vi "enable disable channel for saving.vi"() -> ()   [LabVIEW 2018]
uses:
  <vilib>/Utility/miscctls.llb/LVPointTypeDef.ctl
  <vilib>/Utility/file.llb/Write Delimited Spreadsheet (I64).vi
  <vilib>/Utility/file.llb/Read Delimited Spreadsheet (I64).vi
panel:
  out "size(s) 2":i32=165
  in  "Home Button":bool
  in  "Save Button":bool
  in  "Tab Control":enum32{"Page 1", "Page 2"}(tab)
  in  "Channel 1":cluster{"Enable":bool, "Channel Name":string}={"Enable"=TRUE, "Channel Name"="Time"}
  in  "Channel 2":cluster{"Enable":bool, "Channel Name":string}={"Enable"=TRUE, "Channel Name"="Throttle % "}
  in  "Channel 3":cluster{"Enable":bool, "Channel Name":string}={"Enable"=TRUE, "Channel Name"="Set Speed"}
  in  "Channel 4":cluster{"Enable":bool, "Channel Name":string}={"Enable"=TRUE, "Channel Name"="Speed Summary"}
  in  "Channel 5":cluster{"Enable":bool, "Channel Name":string}={"Enable"=TRUE, "Channel Name"="Torque Summary"}
  in  "Channel 6":cluster{"Enable":bool, "Channel Name":string}={"Enable"=TRUE, "Channel Name"="Power"}
  in  "Channel 7":cluster{"Enable":bool, "Channel Name":string}={"Enable"=TRUE, "Channel Name"="Gear Ratio"}
  in  "Channel 8":cluster{"Enable":bool, "Channel Name":string}={"Enable"=TRUE, "Channel Name"="H Dyno Speed"}
  in  "Channel 9":cluster{"Enable":bool, "Channel Name":string}={"Enable"=TRUE, "Channel Name"="H Dyno Torque"}
  in  "Channel 10":cluster{"Enable":bool, "Channel Name":string}={"Enable"=TRUE, "Channel Name"="L Speed"}
  in  "Channel 11":cluster{"Enable":bool, "Channel Name":string}={"Enable"=TRUE, "Channel Name"="R Speed"}
  in  "Channel 12":cluster{"Enable":bool, "Channel Name":string}={"Enable"=TRUE, "Channel Name"="H Speed"}
  in  "Channel 13":cluster{"Enable":bool, "Channel Name":string}={"Enable"=TRUE, "Channel Name"="L Torque "}
  in  "Channel 14":cluster{"Enable":bool, "Channel Name":string}={"Enable"=TRUE, "Channel Name"="R Torque "}
  in  "Channel 15":cluster{"Enable":bool, "Channel Name":string}={"Enable"=TRUE, "Channel Name"="H Torque "}
  in  "Channel 16":cluster{"Enable":bool, "Channel Name":string}={"Enable"=TRUE, "Channel Name"="T_Oil Gallery"}
  in  "Channel 17":cluster{"Enable":bool, "Channel Name":string}={"Enable"=TRUE, "Channel Name"="T_Coolant_Out"}
  in  "Channel 18":cluster{"Enable":bool, "Channel Name":string}={"Enable"=TRUE, "Channel Name"="T_Coolant_In"}
  in  "Channel 19":cluster{"Enable":bool, "Channel Name":string}={"Enable"=TRUE, "Channel Name"="T_Oil Pan_Out"}
  in  "Channel 20":cluster{"Enable":bool, "Channel Name":string}={"Enable"=TRUE, "Channel Name"="T_Intercooler_In"}
  in  "Channel 21":cluster{"Enable":bool, "Channel Name":string}={"Enable"=TRUE, "Channel Name"="T_Intercooler_Out"}
  in  "Channel 22":cluster{"Enable":bool, "Channel Name":string}={"Enable"=TRUE, "Channel Name"="T_Exhaust_Tail pipe"}
  in  "Channel 23":cluster{"Enable":bool, "Channel Name":string}={"Enable"=TRUE, "Channel Name"="T_frt winding"}
  in  "Channel 24":cluster{"Enable":bool, "Channel Name":string}={"Enable"=TRUE, "Channel Name"="T_Stator Core"}
  in  "Channel 25":cluster{"Enable":bool, "Channel Name":string}={"Enable"=TRUE, "Channel Name"="T_Before Cat"}
  in  "Channel 26":cluster{"Enable":bool, "Channel Name":string}={"Enable"=TRUE, "Channel Name"="TC11"}
  in  "Channel 27":cluster{"Enable":bool, "Channel Name":string}={"Enable"=TRUE, "Channel Name"="TC12"}
  in  "Channel 28":cluster{"Enable":bool, "Channel Name":string}={"Enable"=TRUE, "Channel Name"="TC13"}
  in  "Channel 29":cluster{"Enable":bool, "Channel Name":string}={"Enable"=TRUE, "Channel Name"="TC14"}
  in  "Channel 30":cluster{"Enable":bool, "Channel Name":string}={"Enable"=TRUE, "Channel Name"="TC15"}
  in  "Channel 31":cluster{"Enable":bool, "Channel Name":string}={"Enable"=TRUE, "Channel Name"="TC16"}
  in  "Channel 32":cluster{"Enable":bool, "Channel Name":string}={"Enable"=TRUE, "Channel Name"="P_Oil Gallery"}
  in  "Channel 33":cluster{"Enable":bool, "Channel Name":string}={"Enable"=TRUE, "Channel Name"="P_Coolant_IN"}
  in  "Channel 34":cluster{"Enable":bool, "Channel Name":string}={"Enable"=TRUE, "Channel Name"="P_Coolant_OUT"}
  in  "Channel 35":cluster{"Enable":bool, "Channel Name":string}={"Enable"=TRUE, "Channel Name"="P_Intercooler_In"}
  in  "Channel 36":cluster{"Enable":bool, "Channel Name":string}={"Enable"=TRUE, "Channel Name"="P_Intercooler_out"}
  in  "Channel 37":cluster{"Enable":bool, "Channel Name":string}={"Enable"=TRUE, "Channel Name"="P_Exhaust_TailPipe"}
  in  "Channel 38":cluster{"Enable":bool, "Channel Name":string}={"Enable"=TRUE, "Channel Name"="P_Before cat"}
  in  "Channel 39":cluster{"Enable":bool, "Channel Name":string}={"Enable"=TRUE, "Channel Name"="P_After Air Filter "}
  in  "Channel 40":cluster{"Enable":bool, "Channel Name":string}={"Enable"=TRUE, "Channel Name"="P_Fuel pressure"}
  in  "Channel 41":cluster{"Enable":bool, "Channel Name":string}={"Enable"=TRUE, "Channel Name"="P_CrankCase"}
  in  "Channel 42":cluster{"Enable":bool, "Channel Name":string}={"Enable"=TRUE, "Channel Name"="Spare4"}
  in  "Channel 43":cluster{"Enable":bool, "Channel Name":string}={"Enable"=TRUE, "Channel Name"="Spare5"}
  in  "Channel 44":cluster{"Enable":bool, "Channel Name":string}={"Enable"=TRUE, "Channel Name"="Spare6"}
  in  "Channel 45":cluster{"Enable":bool, "Channel Name":string}={"Enable"=TRUE, "Channel Name"="Spare7"}
  in  "Channel 46":cluster{"Enable":bool, "Channel Name":string}={"Enable"=TRUE, "Channel Name"="Spare8"}
  in  "Channel 47":cluster{"Enable":bool, "Channel Name":string}={"Enable"=TRUE, "Channel Name"="Spare9"}
  in  "Channel 48":cluster{"Enable":bool, "Channel Name":string}={"Enable"=TRUE, "Channel Name"="Ph 1 Voltage"}
  in  "Channel 49":cluster{"Enable":bool, "Channel Name":string}={"Enable"=TRUE, "Channel Name"="Ph 2 Voltage"}
  in  "Channel 50":cluster{"Enable":bool, "Channel Name":string}={"Enable"=TRUE, "Channel Name"="Ph 3 Voltage"}
  in  "Channel 51":cluster{"Enable":bool, "Channel Name":string}={"Enable"=TRUE, "Channel Name"="DC Voltage"}
  in  "Channel 52":cluster{"Enable":bool, "Channel Name":string}={"Enable"=TRUE, "Channel Name"="Votlage 123"}
  in  "Channel 53":cluster{"Enable":bool, "Channel Name":string}={"Enable"=TRUE, "Channel Name"="Ph 1 Current"}
  in  "Channel 54":cluster{"Enable":bool, "Channel Name":string}={"Enable"=TRUE, "Channel Name"="Ph 2 Current"}
  in  "Channel 55":cluster{"Enable":bool, "Channel Name":string}={"Enable"=TRUE, "Channel Name"="Ph 3 Current"}
  in  "Channel 56":cluster{"Enable":bool, "Channel Name":string}={"Enable"=TRUE, "Channel Name"="DC Current"}
  in  "Channel 57":cluster{"Enable":bool, "Channel Name":string}={"Enable"=TRUE, "Channel Name"="Currrent 123"}
  in  "Channel 58":cluster{"Enable":bool, "Channel Name":string}={"Enable"=TRUE, "Channel Name"="Ph 1 power"}
  in  "Channel 59":cluster{"Enable":bool, "Channel Name":string}={"Enable"=TRUE, "Channel Name"="Ph 2 power"}
  in  "Channel 60":cluster{"Enable":bool, "Channel Name":string}={"Enable"=TRUE, "Channel Name"="Ph 3 power"}
  in  "Channel 61":cluster{"Enable":bool, "Channel Name":string}={"Enable"=TRUE, "Channel Name"="DC power"}
  in  "Channel 62":cluster{"Enable":bool, "Channel Name":string}={"Enable"=TRUE, "Channel Name"="P123"}
  in  "Channel 63":cluster{"Enable":bool, "Channel Name":string}={"Enable"=TRUE, "Channel Name"="Ph 1 Freq"}
  in  "Channel 64":cluster{"Enable":bool, "Channel Name":string}={"Enable"=TRUE, "Channel Name"="Ph 2 Freq"}
  in  "Channel 65":cluster{"Enable":bool, "Channel Name":string}={"Enable"=TRUE, "Channel Name"="Ph 3 Freq"}
  in  "Channel 66":cluster{"Enable":bool, "Channel Name":string}={"Enable"=TRUE, "Channel Name"="DesiredSpeedEDriveMfile_20230607"}
  in  "Channel 67":cluster{"Enable":bool, "Channel Name":string}={"Enable"=TRUE, "Channel Name"="DesiredTorqueEDriveMfile_20230607"}
  in  "Channel 68":cluster{"Enable":bool, "Channel Name":string}={"Enable"=TRUE, "Channel Name"="DesiredTorqueDirectionEDriveMfile_20230607"}
  in  "Channel 69":cluster{"Enable":bool, "Channel Name":string}={"Enable"=TRUE, "Channel Name"="Eol_TestFlagEDriveMfile_20230607"}
  in  "Channel 70":cluster{"Enable":bool, "Channel Name":string}={"Enable"=TRUE, "Channel Name"="IdcMaxEDriveMfile_20230607"}
  in  "Channel 71":cluster{"Enable":bool, "Channel Name":string}={"Enable"=TRUE, "Channel Name"="IdcMinEDriveMfile_20230607"}
  in  "Channel 72":cluster{"Enable":bool, "Channel Name":string}={"Enable"=TRUE, "Channel Name"="IsolationStatusEDriveMfile_20230607"}
  in  "Channel 73":cluster{"Enable":bool, "Channel Name":string}={"Enable"=TRUE, "Channel Name"="MainContactorStatusEDriveMfile_20230607"}
  in  "Channel 74":cluster{"Enable":bool, "Channel Name":string}={"Enable"=TRUE, "Channel Name"="OUI_VCU_MCU_CAN_502.MaxSpeedLimitEDriveMfile_20230607"}
  in  "Channel 75":cluster{"Enable":bool, "Channel Name":string}={"Enable"=TRUE, "Channel Name"="MaxTorqueLimitEDriveMfile_20230607"}
  in  "Channel 76":cluster{"Enable":bool, "Channel Name":string}={"Enable"=TRUE, "Channel Name"="OUI_VCU_MCU_CAN_502.MinSpeedLimitEDriveMfile_20230607"}
  in  "Channel 77":cluster{"Enable":bool, "Channel Name":string}={"Enable"=TRUE, "Channel Name"="MinTorqueLimitEDriveMfile_20230607"}
  in  "Channel 78":cluster{"Enable":bool, "Channel Name":string}={"Enable"=TRUE, "Channel Name"="MtrInitAngle_CaliFlagEDriveMfile_20230607"}
  in  "Channel 79":cluster{"Enable":bool, "Channel Name":string}={"Enable"=TRUE, "Channel Name"="RequestedStateINVEDriveMfile_20230607"}
  in  "Channel 80":cluster{"Enable":bool, "Channel Name":string}={"Enable"=TRUE, "Channel Name"="SurgeDamperStateEDriveMfile_20230607"}
  in  "Channel 81":cluster{"Enable":bool, "Channel Name":string}={"Enable"=TRUE, "Channel Name"="UdcMaxEDriveMfile_20230607"}
  in  "Channel 82":cluster{"Enable":bool, "Channel Name":string}={"Enable"=TRUE, "Channel Name"="UdcMinEDriveMfile_20230607"}
  in  "Channel 83":cluster{"Enable":bool, "Channel Name":string}={"Enable"=TRUE, "Channel Name"="BusOffEDriveMfile_20230607"}
  in  "Channel 84":cluster{"Enable":bool, "Channel Name":string}={"Enable"=TRUE, "Channel Name"="Checksum_601EDriveMfile_20230607"}
  in  "Channel 85":cluster{"Enable":bool, "Channel Name":string}={"Enable"=TRUE, "Channel Name"="Checksum_602EDriveMfile_20230607"}
  in  "Channel 86":cluster{"Enable":bool, "Channel Name":string}={"Enable"=TRUE, "Channel Name"="Checksum_606EDriveMfile_20230607"}
  in  "Channel 87":cluster{"Enable":bool, "Channel Name":string}={"Enable"=TRUE, "Channel Name"="ChecksumerrorEDriveMfile_20230607"}
  in  "Channel 88":cluster{"Enable":bool, "Channel Name":string}={"Enable"=TRUE, "Channel Name"="ChecksumwrngEDriveMfile_20230607"}
  in  "Channel 89":cluster{"Enable":bool, "Channel Name":string}={"Enable"=TRUE, "Channel Name"="CurrentHVEDriveMfile_20230607"}
  in  "Channel 90":cluster{"Enable":bool, "Channel Name":string}={"Enable"=TRUE, "Channel Name"="DampTrqEDriveMfile_20230607"}
  in  "Channel 91":cluster{"Enable":bool, "Channel Name":string}={"Enable"=TRUE, "Channel Name"="DamptActiveStateEDriveMfile_20230607"}
  in  "Channel 92":cluster{"Enable":bool, "Channel Name":string}={"Enable"=TRUE, "Channel Name"="DcUOverVWanngEDriveMfile_20230607"}
  in  "Channel 93":cluster{"Enable":bool, "Channel Name":string}={"Enable"=TRUE, "Channel Name"="DcUUnderVWanngEDriveMfile_20230607"}
  in  "Channel 94":cluster{"Enable":bool, "Channel Name":string}={"Enable"=TRUE, "Channel Name"="ElecMotOverSpdWrnngEDriveMfile_20230607"}
  in  "Channel 95":cluster{"Enable":bool, "Channel Name":string}={"Enable"=TRUE, "Channel Name"="ElecMotOverTemWrnngEDriveMfile_20230607"}
  in  "Channel 96":cluster{"Enable":bool, "Channel Name":string}={"Enable"=TRUE, "Channel Name"="ElectricMachineTemperatureEDriveMfile_20230607"}
  in  "Channel 97":cluster{"Enable":bool, "Channel Name":string}={"Enable"=TRUE, "Channel Name"="ErrorCodeEDriveMfile_20230607"}
  in  "Channel 98":cluster{"Enable":bool, "Channel Name":string}={"Enable"=TRUE, "Channel Name"="FaultgradeEDriveMfile_20230607"}
  in  "Channel 99":cluster{"Enable":bool, "Channel Name":string}={"Enable"=TRUE, "Channel Name"="Flt_12V_SnsrHEDriveMfile_20230607"}
  in  "Channel 100":cluster{"Enable":bool, "Channel Name":string}={"Enable"=TRUE, "Channel Name"="Flt_12V_SnsrLEDriveMfile_20230607"}
  in  "Channel 101":cluster{"Enable":bool, "Channel Name":string}={"Enable"=TRUE, "Channel Name"="Flt_CrntSnsrOffset_CompareEDriveMfile_20230607"}
  in  "Channel 102":cluster{"Enable":bool, "Channel Name":string}={"Enable"=TRUE, "Channel Name"="Flt_HW_OVEDriveMfile_20230607"}
  in  "Channel 103":cluster{"Enable":bool, "Channel Name":string}={"Enable"=TRUE, "Channel Name"="Flt_IgbtTem_RampRateEDriveMfile_20230607"}
  in  "Channel 104":cluster{"Enable":bool, "Channel Name":string}={"Enable"=TRUE, "Channel Name"="Flt_IgbtTem_UTEDriveMfile_20230607"}
  in  "Channel 105":cluster{"Enable":bool, "Channel Name":string}={"Enable"=TRUE, "Channel Name"="Flt_IgbtTemp_SampingEDriveMfile_20230607"}
  in  "Channel 106":cluster{"Enable":bool, "Channel Name":string}={"Enable"=TRUE, "Channel Name"="Flt_MessageCounterEDriveMfile_20230607"}
  in  "Channel 107":cluster{"Enable":bool, "Channel Name":string}={"Enable"=TRUE, "Channel Name"="Flt_PhaseCrnt_SumEDriveMfile_20230607"}
  in  "Channel 108":cluster{"Enable":bool, "Channel Name":string}={"Enable"=TRUE, "Channel Name"="Flt_V1p3V_HEDriveMfile_20230607"}
  in  "Channel 109":cluster{"Enable":bool, "Channel Name":string}={"Enable"=TRUE, "Channel Name"="Flt_V1p3V_LEDriveMfile_20230607"}
  in  "Channel 110":cluster{"Enable":bool, "Channel Name":string}={"Enable"=TRUE, "Channel Name"="FluxWeak_FactorEDriveMfile_20230607"}
  in  "Channel 111":cluster{"Enable":bool, "Channel Name":string}={"Enable"=TRUE, "Channel Name"="IGBTOverTemWrnngEDriveMfile_20230607"}
  in  "Channel 112":cluster{"Enable":bool, "Channel Name":string}={"Enable"=TRUE, "Channel Name"="IGBTTemSnsrFltEDriveMfile_20230607"}
  in  "Channel 113":cluster{"Enable":bool, "Channel Name":string}={"Enable"=TRUE, "Channel Name"="INV12VSuppyLVEDriveMfile_20230607"}
  in  "Channel 114":cluster{"Enable":bool, "Channel Name":string}={"Enable"=TRUE, "Channel Name"="INV12VSuppyOVEDriveMfile_20230607"}
  in  "Channel 115":cluster{"Enable":bool, "Channel Name":string}={"Enable"=TRUE, "Channel Name"="INV15VSuppyLVEDriveMfile_20230607"}
  in  "Channel 116":cluster{"Enable":bool, "Channel Name":string}={"Enable"=TRUE, "Channel Name"="INV15VSuppyOVEDriveMfile_20230607"}
  in  "Channel 117":cluster{"Enable":bool, "Channel Name":string}={"Enable"=TRUE, "Channel Name"="INV5VSuppyLVEDriveMfile_20230607"}
  in  "Channel 118":cluster{"Enable":bool, "Channel Name":string}={"Enable"=TRUE, "Channel Name"="INV5VSuppyOVEDriveMfile_20230607"}
  in  "Channel 119":cluster{"Enable":bool, "Channel Name":string}={"Enable"=TRUE, "Channel Name"="INVDschrgFltEDriveMfile_20230607"}
  in  "Channel 120":cluster{"Enable":bool, "Channel Name":string}={"Enable"=TRUE, "Channel Name"="INVOverVolFltEDriveMfile_20230607"}
  in  "Channel 121":cluster{"Enable":bool, "Channel Name":string}={"Enable"=TRUE, "Channel Name"="INVPwrModuFltEDriveMfile_20230607"}
  in  "Channel 122":cluster{"Enable":bool, "Channel Name":string}={"Enable"=TRUE, "Channel Name"="INVVolSnsrFltEDriveMfile_20230607"}
  in  "Channel 123":cluster{"Enable":bool, "Channel Name":string}={"Enable"=TRUE, "Channel Name"="Id_FBEDriveMfile_20230607"}
  in  "Channel 124":cluster{"Enable":bool, "Channel Name":string}={"Enable"=TRUE, "Channel Name"="Id_RefEDriveMfile_20230607"}
  in  "Channel 125":cluster{"Enable":bool, "Channel Name":string}={"Enable"=TRUE, "Channel Name"="InitAngleOffsetEDriveMfile_20230607"}
  in  "Channel 126":cluster{"Enable":bool, "Channel Name":string}={"Enable"=TRUE, "Channel Name"="InverterTemperatureEDriveMfile_20230607"}
  in  "Channel 127":cluster{"Enable":bool, "Channel Name":string}={"Enable"=TRUE, "Channel Name"="Iq_FBEDriveMfile_20230607"}
  in  "Channel 128":cluster{"Enable":bool, "Channel Name":string}={"Enable"=TRUE, "Channel Name"="Iq_RefEDriveMfile_20230607"}
  in  "Channel 129":cluster{"Enable":bool, "Channel Name":string}={"Enable"=TRUE, "Channel Name"="LostCommWithVCUEDriveMfile_20230607"}
  in  "Channel 130":cluster{"Enable":bool, "Channel Name":string}={"Enable"=TRUE, "Channel Name"="MCU_InitialErrEDriveMfile_20230607"}
  in  "Channel 131":cluster{"Enable":bool, "Channel Name":string}={"Enable"=TRUE, "Channel Name"="MaxTorqueEDriveMfile_20230607"}
  in  "Channel 132":cluster{"Enable":bool, "Channel Name":string}={"Enable"=TRUE, "Channel Name"="MessageCounter_606EDriveMfile_20230607"}
  in  "Channel 133":cluster{"Enable":bool, "Channel Name":string}={"Enable"=TRUE, "Channel Name"="MinTorqueEDriveMfile_20230607"}
  in  "Channel 134":cluster{"Enable":bool, "Channel Name":string}={"Enable"=TRUE, "Channel Name"="MotOverCrntFltEDriveMfile_20230607"}
  in  "Channel 135":cluster{"Enable":bool, "Channel Name":string}={"Enable"=TRUE, "Channel Name"="MotOverCrntFltHardEDriveMfile_20230607"}
  in  "Channel 136":cluster{"Enable":bool, "Channel Name":string}={"Enable"=TRUE, "Channel Name"="MotOverSpdFltEDriveMfile_20230607"}
  in  "Channel 137":cluster{"Enable":bool, "Channel Name":string}={"Enable"=TRUE, "Channel Name"="MotOverTemFltEDriveMfile_20230607"}
  in  "Channel 138":cluster{"Enable":bool, "Channel Name":string}={"Enable"=TRUE, "Channel Name"="MotRotBlockFltEDriveMfile_20230607"}
  in  "Channel 139":cluster{"Enable":bool, "Channel Name":string}={"Enable"=TRUE, "Channel Name"="MotRsovrFltEDriveMfile_20230607"}
  in  "Channel 140":cluster{"Enable":bool, "Channel Name":string}={"Enable"=TRUE, "Channel Name"="MotTemSnsrFltEDriveMfile_20230607"}
  in  "Channel 141":cluster{"Enable":bool, "Channel Name":string}={"Enable"=TRUE, "Channel Name"="MtrSpdFilt_NoFiltEDriveMfile_20230607"}
  in  "Channel 142":cluster{"Enable":bool, "Channel Name":string}={"Enable"=TRUE, "Channel Name"="OutputSpeedEDriveMfile_20230607"}
  in  "Channel 143":cluster{"Enable":bool, "Channel Name":string}={"Enable"=TRUE, "Channel Name"="OutputTorqueEDriveMfile_20230607"}
  in  "Channel 144":cluster{"Enable":bool, "Channel Name":string}={"Enable"=TRUE, "Channel Name"="PhaseACrntSnsrFltEDriveMfile_20230607"}
  in  "Channel 145":cluster{"Enable":bool, "Channel Name":string}={"Enable"=TRUE, "Channel Name"="PhaseBCrntSnsrFltEDriveMfile_20230607"}
  in  "Channel 146":cluster{"Enable":bool, "Channel Name":string}={"Enable"=TRUE, "Channel Name"="PhaseCCrntSnsrFltEDriveMfile_20230607"}
  in  "Channel 147":cluster{"Enable":bool, "Channel Name":string}={"Enable"=TRUE, "Channel Name"="PowerEDriveMfile_20230607"}
  in  "Channel 148":cluster{"Enable":bool, "Channel Name":string}={"Enable"=TRUE, "Channel Name"="SW_EditionEDriveMfile_20230607"}
  in  "Channel 149":cluster{"Enable":bool, "Channel Name":string}={"Enable"=TRUE, "Channel Name"="StateEDriveMfile_20230607"}
  in  "Channel 150":cluster{"Enable":bool, "Channel Name":string}={"Enable"=TRUE, "Channel Name"="TrqRefFnlEDriveMfile_20230607"}
  in  "Channel 151":cluster{"Enable":bool, "Channel Name":string}={"Enable"=TRUE, "Channel Name"="Ud_RefEDriveMfile_20230607"}
  in  "Channel 152":cluster{"Enable":bool, "Channel Name":string}={"Enable"=TRUE, "Channel Name"="Uq_RefEDriveMfile_20230607"}
  in  "Channel 153":cluster{"Enable":bool, "Channel Name":string}={"Enable"=TRUE, "Channel Name"="VoltUsageEDriveMfile_20230607"}
  in  "Channel 154":cluster{"Enable":bool, "Channel Name":string}={"Enable"=TRUE, "Channel Name"="VoltageHVEDriveMfile_20230607"}
  in  "Channel 155":cluster{"Enable":bool, "Channel Name":string}={"Enable"=TRUE, "Channel Name"="War_IgbtTem_UTEDriveMfile_20230607"}
  in  "Channel 156":cluster{"Enable":bool, "Channel Name":string}={"Enable"=TRUE, "Channel Name"="War_MtrTem_UTEDriveMfile_20230607"}
  in  "Channel 157":cluster{"Enable":bool, "Channel Name":string}={"Enable"=TRUE, "Channel Name"="War_PhaseOverCrntEDriveMfile_20230607"}
  in  "Channel 158":cluster{"Enable":bool, "Channel Name":string}={"Enable"=TRUE, "Channel Name"="phaseA_currentEDriveMfile_20230607"}
  in  "Channel 159":cluster{"Enable":bool, "Channel Name":string}={"Enable"=TRUE, "Channel Name"="phaseB_currentEDriveMfile_20230607"}
  in  "Channel 160":cluster{"Enable":bool, "Channel Name":string}={"Enable"=TRUE, "Channel Name"="phaseC_currentEDriveMfile_20230607"}
  in  "Channel 161":cluster{"Enable":bool, "Channel Name":string}={"Enable"=TRUE, "Channel Name"="HVHC SELECTION"}
  in  "Channel 162":cluster{"Enable":bool, "Channel Name":string}={"Enable"=TRUE, "Channel Name"="CONTROL SELECTION"}
  in  "Channel 163":cluster{"Enable":bool, "Channel Name":string}={"Enable"=TRUE, "Channel Name"="VOLTAGE"}
  in  "Channel 164":cluster{"Enable":bool, "Channel Name":string}={"Enable"=TRUE, "Channel Name"="CURRENT"}
  in  "Channel 165":cluster{"Enable":bool, "Channel Name":string}={"Enable"=TRUE, "Channel Name"="POWER"}
  in  "Channel 166":cluster{"Enable":bool, "Channel Name":string}={"Enable"=TRUE, "Channel Name"=""}
  in  "Channel 167":cluster{"Enable":bool, "Channel Name":string}={"Enable"=TRUE, "Channel Name"=""}
  in  "Channel 168":cluster{"Enable":bool, "Channel Name":string}={"Enable"=TRUE, "Channel Name"=""}
  out "size(s)":i32=165
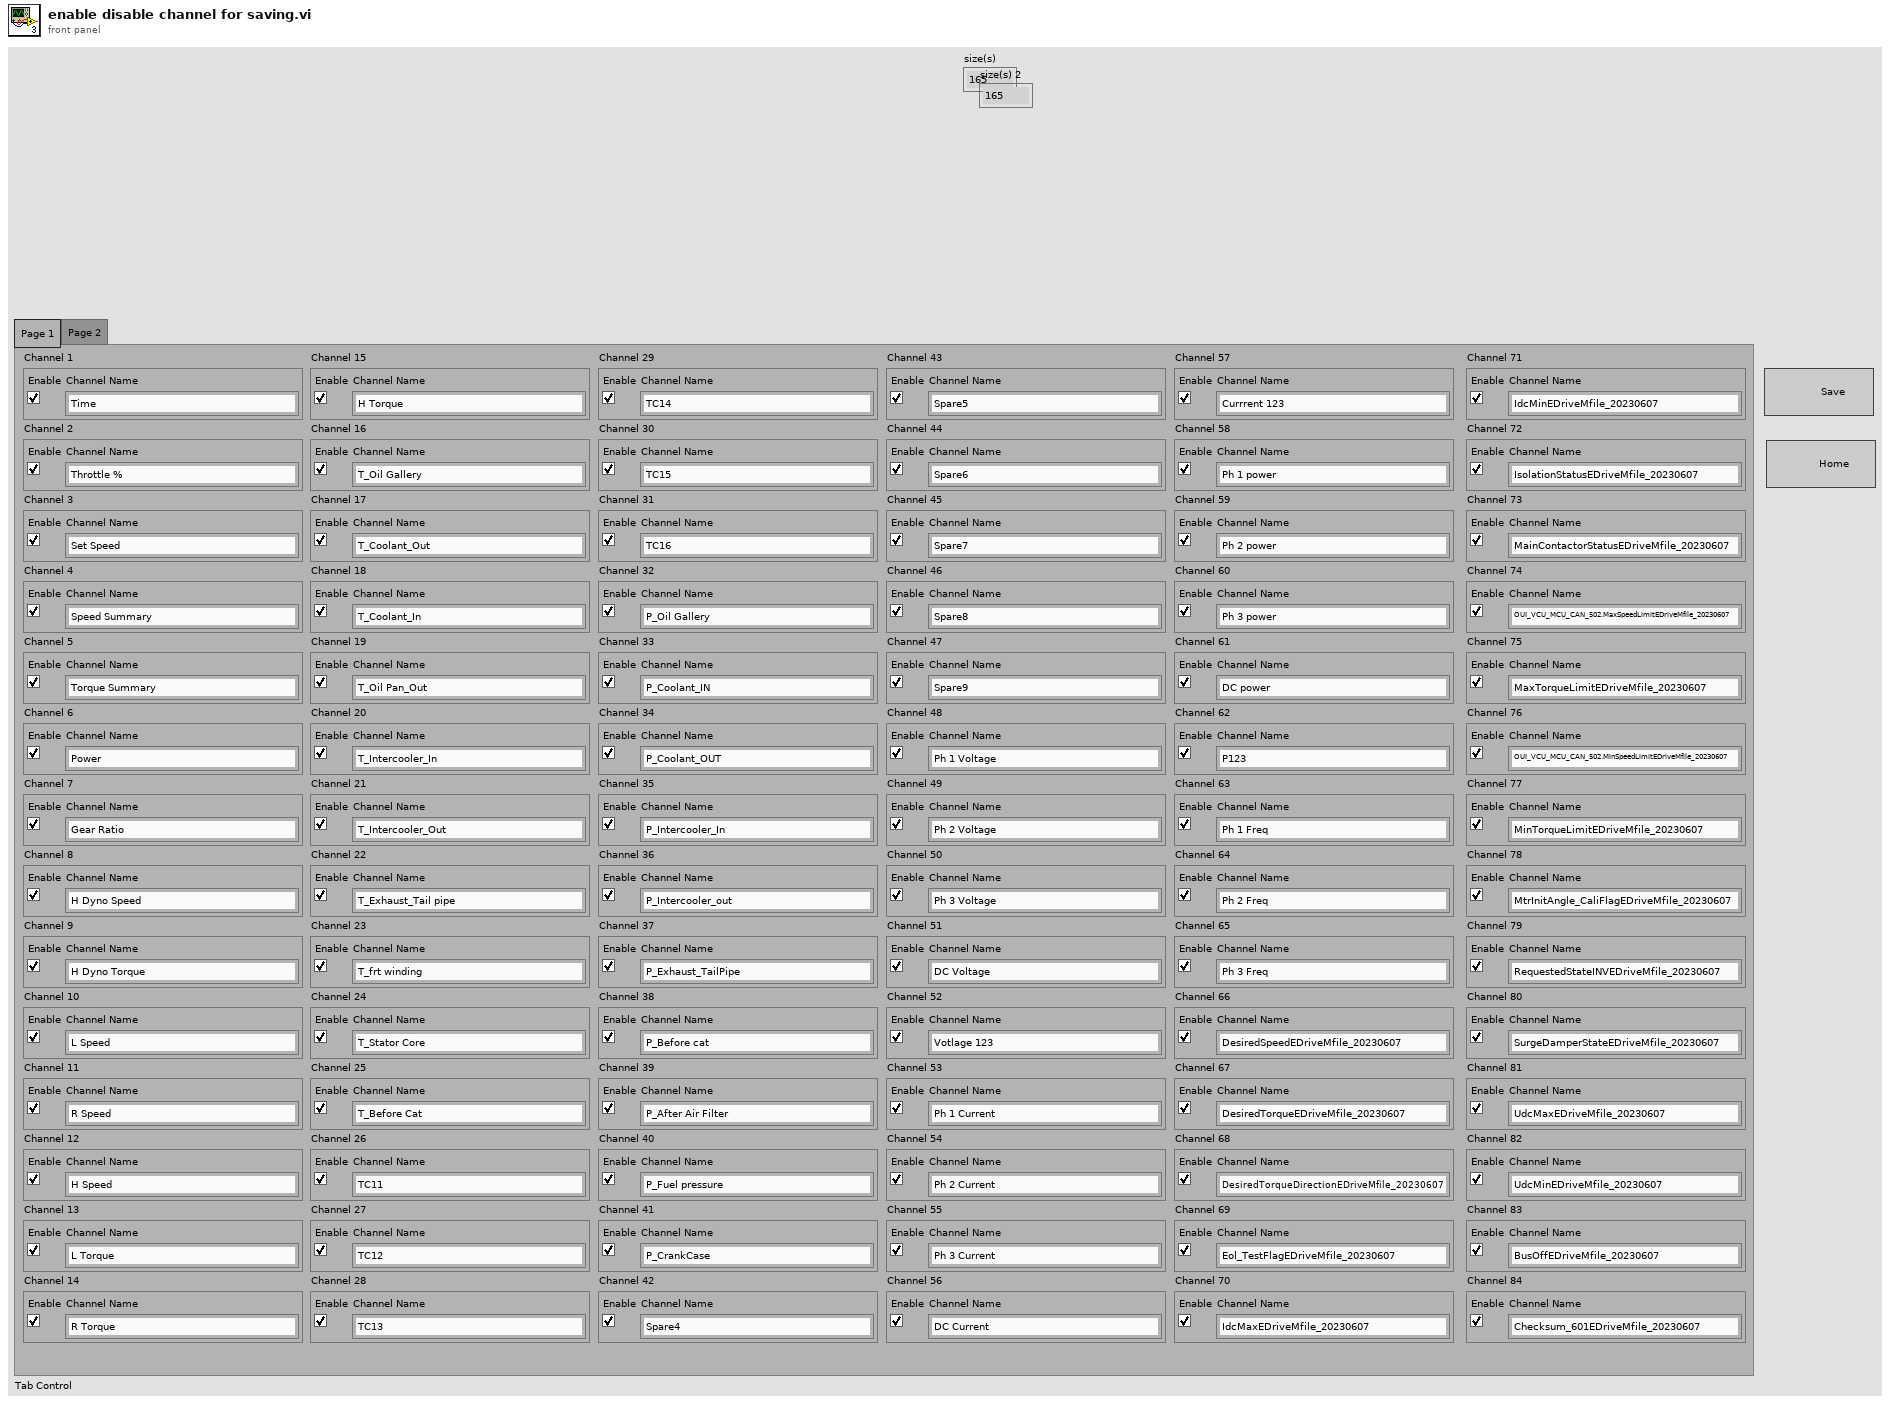
[diagram p1: front panel]
types:
  T1 = typedef "LVPointTypeDef.ctl" = cluster{"Horizontal":i16, "Vertical":i16}
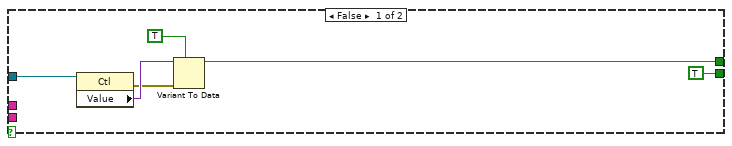
[diagram p3: hidden frame]
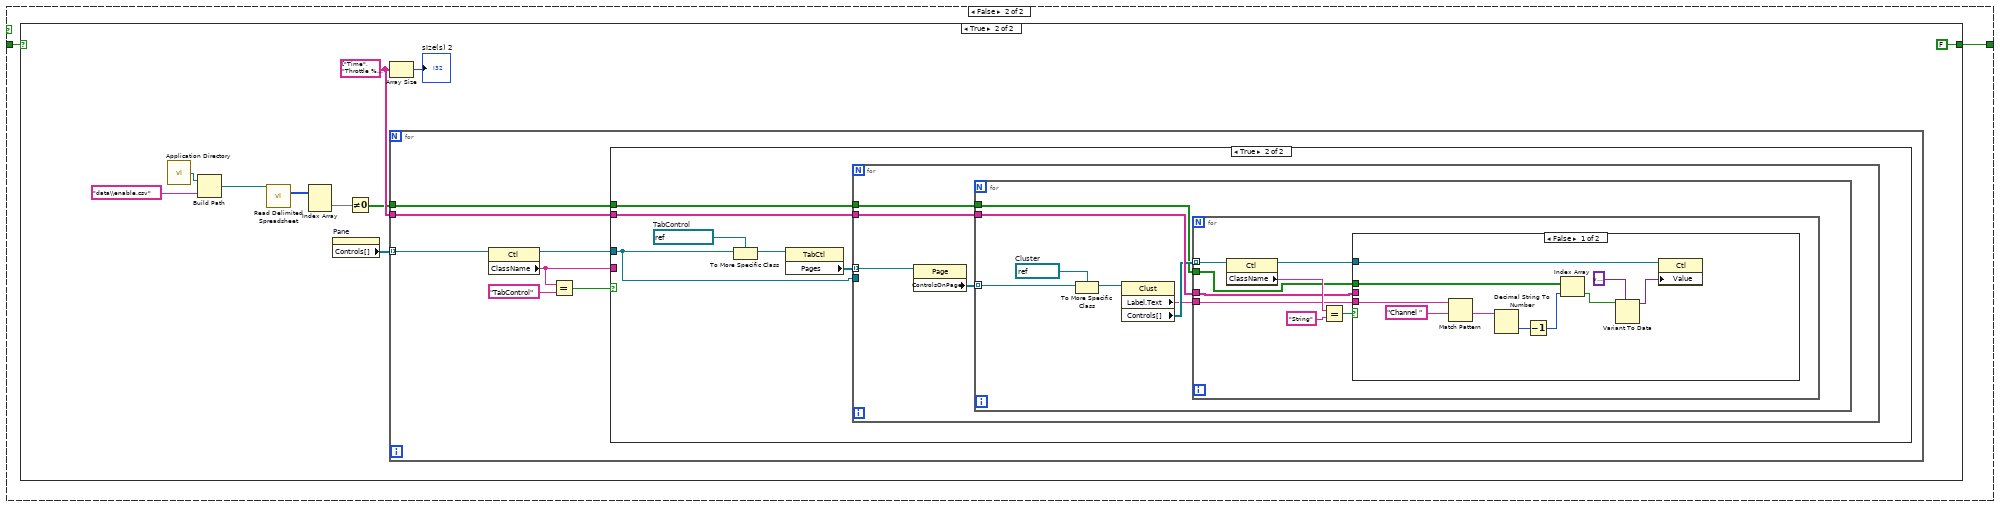
[diagram p5: hidden frame]
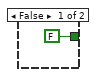
[diagram p6: hidden frame]
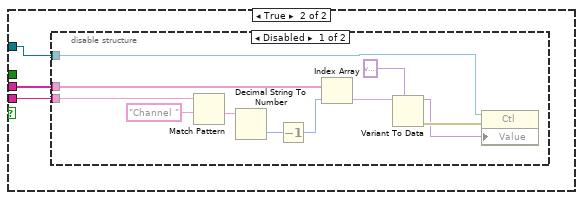
[diagram p8: hidden frame]
diagram:
  n1 = property on="Pane" class="Pane"("Origin"=T1 {"Horizontal"=0, "Vertical"=0}) -> (error out=w1:errorcluster)  [unwired: 2 in, 1 out]
  n2 = while {
    shift-right: [w4] -> _
    shift-left: TRUE -> [w5]
    tunnel: w1 -> [_]
    stop <- "Home Button" stop-if-true
    n3 = Wait (ms)(milliseconds to wait=u32 500) -> ()  [unwired: 1 out]
    n4 = case shown="True" "Save Button" {
      tunnel: w5 -> [w9 w75]
      tunnel: [w9 w74] -> w4
      frame True {
        w16 = string[] ["Time", "Throttle % ", "Set Speed", "Speed Summary", "Torque Summary", "Power", "Gear Ratio", "H Dyno Speed", "H Dyno Torque", "L Speed", "R Speed", "H Speed", "L Torque ", "R Torque ", "H Torque ", "T_Oil Gallery", "T_Coolant_Out", "T_Coolant_In", "T_Oil Pan_Out", "T_Intercooler_In", "T_Intercooler_Out", "T_Exhaust_Tail pipe", "T_frt winding", "T_Stator Core", "T_Before Cat", "TC11", "TC12", "TC13", "TC14", "TC15", "TC16", "P_Oil Gallery", "P_Coolant_IN", "P_Coolant_OUT", "P_Intercooler_In", "P_Intercooler_out", "P_Exhaust_TailPipe", "P_Before cat", "P_After Air Filter ", "P_Fuel pressure", "P_CrankCase", "Spare4", "Spare5", "Spare6", "Spare7", "Spare8", "Spare9", "Ph 1 Voltage", "Ph 2 Voltage", "Ph 3 Voltage", "DC Voltage", "Votlage 123", "Ph 1 Current", "Ph 2 Current", "Ph 3 Current", "DC Current", "Currrent 123", "Ph 1 power", "Ph 2 power", "Ph 3 power", "DC power", "P123", "Ph 1 Freq", "Ph 2 Freq", "Ph 3 Freq", "DesiredSpeedEDriveMfile_20230607", "DesiredTorqueEDriveMfile_20230607", "DesiredTorqueDirectionEDriveMfile_20230607", "Eol_TestFlagEDriveMfile_20230607", "IdcMaxEDriveMfile_20230607", "IdcMinEDriveMfile_20230607", "IsolationStatusEDriveMfile_20230607", "MainContactorStatusEDriveMfile_20230607", "OUI_VCU_MCU_CAN_502.MaxSpeedLimitEDriveMfile_20230607", "MaxTorqueLimitEDriveMfile_20230607", "OUI_VCU_MCU_CAN_502.MinSpeedLimitEDriveMfile_20230607", "MinTorqueLimitEDriveMfile_20230607", "MtrInitAngle_CaliFlagEDriveMfile_20230607", "RequestedStateINVEDriveMfile_20230607", "SurgeDamperStateEDriveMfile_20230607", "UdcMaxEDriveMfile_20230607", "UdcMinEDriveMfile_20230607", "BusOffEDriveMfile_20230607", "Checksum_601EDriveMfile_20230607", "Checksum_602EDriveMfile_20230607", "Checksum_606EDriveMfile_20230607", "ChecksumerrorEDriveMfile_20230607", "ChecksumwrngEDriveMfile_20230607", "CurrentHVEDriveMfile_20230607", "DampTrqEDriveMfile_20230607", "DamptActiveStateEDriveMfile_20230607", "DcUOverVWanngEDriveMfile_20230607", "DcUUnderVWanngEDriveMfile_20230607", "ElecMotOverSpdWrnngEDriveMfile_20230607", "ElecMotOverTemWrnngEDriveMfile_20230607", "ElectricMachineTemperatureEDriveMfile_20230607", "ErrorCodeEDriveMfile_20230607", "FaultgradeEDriveMfile_20230607", "Flt_12V_SnsrHEDriveMfile_20230607", "Flt_12V_SnsrLEDriveMfile_20230607", "Flt_CrntSnsrOffset_CompareEDriveMfile_20230607", "Flt_HW_OVEDriveMfile_20230607", "Flt_IgbtTem_RampRateEDriveMfile_20230607", "Flt_IgbtTem_UTEDriveMfile_20230607", "Flt_IgbtTemp_SampingEDriveMfile_20230607", "Flt_MessageCounterEDriveMfile_20230607", "Flt_PhaseCrnt_SumEDriveMfile_20230607", "Flt_V1p3V_HEDriveMfile_20230607", "Flt_V1p3V_LEDriveMfile_20230607", "FluxWeak_FactorEDriveMfile_20230607", "IGBTOverTemWrnngEDriveMfile_20230607", "IGBTTemSnsrFltEDriveMfile_20230607", "INV12VSuppyLVEDriveMfile_20230607", "INV12VSuppyOVEDriveMfile_20230607", "INV15VSuppyLVEDriveMfile_20230607", "INV15VSuppyOVEDriveMfile_20230607", "INV5VSuppyLVEDriveMfile_20230607", "INV5VSuppyOVEDriveMfile_20230607", "INVDschrgFltEDriveMfile_20230607", "INVOverVolFltEDriveMfile_20230607", "INVPwrModuFltEDriveMfile_20230607", "INVVolSnsrFltEDriveMfile_20230607", "Id_FBEDriveMfile_20230607", "Id_RefEDriveMfile_20230607", "InitAngleOffsetEDriveMfile_20230607", "InverterTemperatureEDriveMfile_20230607", "Iq_FBEDriveMfile_20230607", "Iq_RefEDriveMfile_20230607", "LostCommWithVCUEDriveMfile_20230607", "MCU_InitialErrEDriveMfile_20230607", "MaxTorqueEDriveMfile_20230607", "MessageCounter_606EDriveMfile_20230607", "MinTorqueEDriveMfile_20230607", "MotOverCrntFltEDriveMfile_20230607", "MotOverCrntFltHardEDriveMfile_20230607", "MotOverSpdFltEDriveMfile_20230607", "MotOverTemFltEDriveMfile_20230607", "MotRotBlockFltEDriveMfile_20230607", "MotRsovrFltEDriveMfile_20230607", "MotTemSnsrFltEDriveMfile_20230607", "MtrSpdFilt_NoFiltEDriveMfile_20230607", "OutputSpeedEDriveMfile_20230607", "OutputTorqueEDriveMfile_20230607", "PhaseACrntSnsrFltEDriveMfile_20230607", "PhaseBCrntSnsrFltEDriveMfile_20230607", "PhaseCCrntSnsrFltEDriveMfile_20230607", "PowerEDriveMfile_20230607", "SW_EditionEDriveMfile_20230607", "StateEDriveMfile_20230607", "TrqRefFnlEDriveMfile_20230607", "Ud_RefEDriveMfile_20230607", "Uq_RefEDriveMfile_20230607", "VoltUsageEDriveMfile_20230607", "VoltageHVEDriveMfile_20230607", "War_IgbtTem_UTEDriveMfile_20230607", "War_MtrTem_UTEDriveMfile_20230607", "War_PhaseOverCrntEDriveMfile_20230607", "phaseA_currentEDriveMfile_20230607", "phaseB_currentEDriveMfile_20230607", "phaseC_currentEDriveMfile_20230607", "HVHC SELECTION", "CONTROL SELECTION", "VOLTAGE", "CURRENT", "POWER"] ("deleted portion")
        n5 = property on="Pane" class="Pane"() -> ("Controls[]"=w17:refnum<vi>[])  [unwired: 2 in, 2 out]
        n6 = for {
          tunnel: w17 -> [w26] mode=indexing
          tunnel: w16 -> [w25]
          tunnel: [w20] -> w15 mode=concatenating if=w19
          n7 = property class="Ctl"(reference=w26) -> (reference out=w22:refnum<vi>, "ClassName"=w23:string)  [unwired: 1 in, 1 out]
          n8 = Equal?(x=w23, y="TabControl") -> (x = y?=w21:bool)
          n9 = case shown="True" w21 {
            tunnel: w25 -> [_ w33]
            tunnel: w23 -> [_ _]
            tunnel: w22 -> [_ w31]
            tunnel: [_ w28] -> w20
            tunnel: [_ TRUE] -> w19
            frame False {
            }
            frame True {
              w32 = refnum<vi> refnum  # TabControl
              n10 = To More Specific Class(target class=w32, reference=w31) -> (specific class reference=w30:refnum<vi>)  [unwired: 1 in, 1 out]
              n11 = property class="TabCtl"(reference=w30) -> ("Pages"=w29:refnum<vi>[])  [unwired: 1 in, 2 out]
              n12 = for {
                tunnel: w33 -> [w37]
                tunnel: w31 -> [_]
                tunnel: w29 -> [w36] mode=indexing
                tunnel: [w34] -> w28 mode=concatenating
                n13 = property class="Page"(reference=w36) -> ("ControlsOnPage"=w35:refnum<vi>[])  [unwired: 1 in, 2 out]
                n14 = for {
                  tunnel: w37 -> [w44]
                  tunnel: w35 -> [w43] mode=indexing
                  tunnel: [w38] -> w34 mode=concatenating
                  w42 = refnum<vi> refnum  # Cluster
                  n15 = To More Specific Class(target class=w42, reference=w43) -> (specific class reference=w41:refnum<vi>)  [unwired: 1 in, 1 out]
                  n16 = property class="Clust"(reference=w41) -> ("Label.Text"=w39:string, "Controls[]"=w40:refnum<vi>[])  [unwired: 1 in, 2 out]
                  n17 = for {
                    tunnel: w40 -> [w51] mode=indexing
                    tunnel: w39 -> [w48]
                    tunnel: w44 -> [w47]
                    tunnel: [w46] -> w38 mode=indexing if=w45
                    n18 = property class="Ctl"(reference=w51) -> (reference out=w49:refnum<vi>, "ClassName"=w52:string)  [unwired: 1 in, 1 out]
                    n19 = Equal?(x=w52, y="String") -> (x = y?=w50:bool)
                    n20 = case shown="True" w50 {
                      tunnel: w49 -> [w59 w62]
                      tunnel: w48 -> [_ w61]
                      tunnel: w47 -> [_ w60]
                      tunnel: [w55 _] -> w46
                      tunnel: [TRUE _] -> w45
                      frame False {
                        n21 = property class="Ctl"(reference=w59) -> (error out=w56:errorcluster, "Value"=w58:variant)  [unwired: 1 in, 1 out]
                        n22 = Variant To Data(error in=w56, type=TRUE, Variant=w58) -> (data=w55:bool)  [unwired: 1 out]
                      }
                      frame True {
                        n23 = disable-structure shown="Disabled" {
                          disable-tunnel: w62 -> [w73 _]
                          disable-tunnel: w61 -> [w72 _]
                          disable-tunnel: w60 -> [w71 _]
                          frame Disabled {
                            n24 = Match Pattern(string=w72, regular expression="Channel ") -> (after substring=w69:string)  [unwired: 1 in, 3 out]
                            n25 = Decimal String To Number(string=w69) -> (number=w68:i32)  [unwired: 2 in, 1 out]
                            n26 = Decrement(x=w68) -> (x-1=w67:i32)
                            n27 = Index Array(array=w71, index=w67) -> (element=w66:string)
                            n28 = Variant To Data(type=variant ("Value"), Variant=w66) -> (data=w63:variant, error out=w64:errorcluster)  [unwired: 1 in]
                            n29 = property class="Ctl"(reference=w73, error in=w64, "Value"=w63) -> ()  [unwired: 2 out]
                          }
                          frame Enabled {
                          }
                        }
                      }
                    }
                  }
                }
              }
            }
          }
        }
        n30 = Array Size(array=w16) -> (size(s)=→"size(s)":i32)
        n31 = call <vilib>:"Application Directory.vi"() -> ("Application Directory"=w12:path)
        n32 = Build Array(w15) -> (w14:bool[][])
        n33 = Build Path(base path=w12, name or relative path="data\\enable.csv") -> (appended path=w10:path)
        n34 = Boolean To (0,1)(Boolean=w14) -> (0, 1=w13:i16[][])
        n35 = call-poly <vilib>:"Write Delimited Spreadsheet.vi"("file path (dialog if empty)"=w10, "2D data"=w13) -> ()  [unwired: 12 in, 2 out]
      }
      frame False {
        n36 = case shown="True" w75 {
          tunnel: [FALSE FALSE] -> w74
          frame False {
          }
          frame True {
            w84 = string[] ["Time", "Throttle % ", "Set Speed", "Speed Summary", "Torque Summary", "Power", "Gear Ratio", "H Dyno Speed", "H Dyno Torque", "L Speed", "R Speed", "H Speed", "L Torque ", "R Torque ", "H Torque ", "T_Oil Gallery", "T_Coolant_Out", "T_Coolant_In", "T_Oil Pan_Out", "T_Intercooler_In", "T_Intercooler_Out", "T_Exhaust_Tail pipe", "T_frt winding", "T_Stator Core", "T_Before Cat", "TC11", "TC12", "TC13", "TC14", "TC15", "TC16", "P_Oil Gallery", "P_Coolant_IN", "P_Coolant_OUT", "P_Intercooler_In", "P_Intercooler_out", "P_Exhaust_TailPipe", "P_Before cat", "P_After Air Filter ", "P_Fuel pressure", "P_CrankCase", "Spare4", "Spare5", "Spare6", "Spare7", "Spare8", "Spare9", "Ph 1 Voltage", "Ph 2 Voltage", "Ph 3 Voltage", "DC Voltage", "Votlage 123", "Ph 1 Current", "Ph 2 Current", "Ph 3 Current", "DC Current", "Currrent 123", "Ph 1 power", "Ph 2 power", "Ph 3 power", "DC power", "P123", "Ph 1 Freq", "Ph 2 Freq", "Ph 3 Freq", "DesiredSpeedEDriveMfile_20230607", "DesiredTorqueEDriveMfile_20230607", "DesiredTorqueDirectionEDriveMfile_20230607", "Eol_TestFlagEDriveMfile_20230607", "IdcMaxEDriveMfile_20230607", "IdcMinEDriveMfile_20230607", "IsolationStatusEDriveMfile_20230607", "MainContactorStatusEDriveMfile_20230607", "OUI_VCU_MCU_CAN_502.MaxSpeedLimitEDriveMfile_20230607", "MaxTorqueLimitEDriveMfile_20230607", "OUI_VCU_MCU_CAN_502.MinSpeedLimitEDriveMfile_20230607", "MinTorqueLimitEDriveMfile_20230607", "MtrInitAngle_CaliFlagEDriveMfile_20230607", "RequestedStateINVEDriveMfile_20230607", "SurgeDamperStateEDriveMfile_20230607", "UdcMaxEDriveMfile_20230607", "UdcMinEDriveMfile_20230607", "BusOffEDriveMfile_20230607", "Checksum_601EDriveMfile_20230607", "Checksum_602EDriveMfile_20230607", "Checksum_606EDriveMfile_20230607", "ChecksumerrorEDriveMfile_20230607", "ChecksumwrngEDriveMfile_20230607", "CurrentHVEDriveMfile_20230607", "DampTrqEDriveMfile_20230607", "DamptActiveStateEDriveMfile_20230607", "DcUOverVWanngEDriveMfile_20230607", "DcUUnderVWanngEDriveMfile_20230607", "ElecMotOverSpdWrnngEDriveMfile_20230607", "ElecMotOverTemWrnngEDriveMfile_20230607", "ElectricMachineTemperatureEDriveMfile_20230607", "ErrorCodeEDriveMfile_20230607", "FaultgradeEDriveMfile_20230607", "Flt_12V_SnsrHEDriveMfile_20230607", "Flt_12V_SnsrLEDriveMfile_20230607", "Flt_CrntSnsrOffset_CompareEDriveMfile_20230607", "Flt_HW_OVEDriveMfile_20230607", "Flt_IgbtTem_RampRateEDriveMfile_20230607", "Flt_IgbtTem_UTEDriveMfile_20230607", "Flt_IgbtTemp_SampingEDriveMfile_20230607", "Flt_MessageCounterEDriveMfile_20230607", "Flt_PhaseCrnt_SumEDriveMfile_20230607", "Flt_V1p3V_HEDriveMfile_20230607", "Flt_V1p3V_LEDriveMfile_20230607", "FluxWeak_FactorEDriveMfile_20230607", "IGBTOverTemWrnngEDriveMfile_20230607", "IGBTTemSnsrFltEDriveMfile_20230607", "INV12VSuppyLVEDriveMfile_20230607", "INV12VSuppyOVEDriveMfile_20230607", "INV15VSuppyLVEDriveMfile_20230607", "INV15VSuppyOVEDriveMfile_20230607", "INV5VSuppyLVEDriveMfile_20230607", "INV5VSuppyOVEDriveMfile_20230607", "INVDschrgFltEDriveMfile_20230607", "INVOverVolFltEDriveMfile_20230607", "INVPwrModuFltEDriveMfile_20230607", "INVVolSnsrFltEDriveMfile_20230607", "Id_FBEDriveMfile_20230607", "Id_RefEDriveMfile_20230607", "InitAngleOffsetEDriveMfile_20230607", "InverterTemperatureEDriveMfile_20230607", "Iq_FBEDriveMfile_20230607", "Iq_RefEDriveMfile_20230607", "LostCommWithVCUEDriveMfile_20230607", "MCU_InitialErrEDriveMfile_20230607", "MaxTorqueEDriveMfile_20230607", "MessageCounter_606EDriveMfile_20230607", "MinTorqueEDriveMfile_20230607", "MotOverCrntFltEDriveMfile_20230607", "MotOverCrntFltHardEDriveMfile_20230607", "MotOverSpdFltEDriveMfile_20230607", "MotOverTemFltEDriveMfile_20230607", "MotRotBlockFltEDriveMfile_20230607", "MotRsovrFltEDriveMfile_20230607", "MotTemSnsrFltEDriveMfile_20230607", "MtrSpdFilt_NoFiltEDriveMfile_20230607", "OutputSpeedEDriveMfile_20230607", "OutputTorqueEDriveMfile_20230607", "PhaseACrntSnsrFltEDriveMfile_20230607", "PhaseBCrntSnsrFltEDriveMfile_20230607", "PhaseCCrntSnsrFltEDriveMfile_20230607", "PowerEDriveMfile_20230607", "SW_EditionEDriveMfile_20230607", "StateEDriveMfile_20230607", "TrqRefFnlEDriveMfile_20230607", "Ud_RefEDriveMfile_20230607", "Uq_RefEDriveMfile_20230607", "VoltUsageEDriveMfile_20230607", "VoltageHVEDriveMfile_20230607", "War_IgbtTem_UTEDriveMfile_20230607", "War_MtrTem_UTEDriveMfile_20230607", "War_PhaseOverCrntEDriveMfile_20230607", "phaseA_currentEDriveMfile_20230607", "phaseB_currentEDriveMfile_20230607", "phaseC_currentEDriveMfile_20230607", "HVHC SELECTION", "CONTROL SELECTION", "VOLTAGE", "CURRENT", "POWER"] ("deleted portion")
            n37 = call <vilib>:"Application Directory.vi"() -> ("Application Directory"=w83:path)
            n38 = Build Path(base path=w83, name or relative path="data\\enable.csv") -> (appended path=w81:path)
            n39 = call-poly <vilib>:"Read Delimited Spreadsheet.vi"("file path (dialog if empty)"=w81) -> ("all rows"=w80:i64[][])  [unwired: 9 in, 5 out]
            n40 = Index Array(array=w80) -> (element=w79:i64[])  [unwired: 2 in]
            n41 = property on="Pane" class="Pane"() -> ("Controls[]"=w85:refnum<vi>[])  [unwired: 2 in, 2 out]
            n42 = Not Equal To 0?(x=w79) -> (x != 0?=w78:bool[])
            n43 = Array Size(array=w84) -> (size(s)=→"size(s) 2":i32)
            n44 = for {
              tunnel: w85 -> [w93] mode=indexing
              tunnel: w84 -> [w92]
              tunnel: w78 -> [w87]
              n45 = property class="Ctl"(reference=w93) -> (reference out=w89:refnum<vi>, "ClassName"=w90:string)  [unwired: 1 in, 1 out]
              n46 = Equal?(x=w90, y="TabControl") -> (x = y?=w88:bool)
              n47 = case shown="True" w88 {
                tunnel: w92 -> [_ w99]
                tunnel: w90 -> [_ _]
                tunnel: w89 -> [_ w97]
                tunnel: w87 -> [_ w94]
                frame False {
                }
                frame True {
                  w98 = refnum<vi> refnum  # TabControl
                  n48 = To More Specific Class(target class=w98, reference=w97) -> (specific class reference=w96:refnum<vi>)  [unwired: 1 in, 1 out]
                  n49 = property class="TabCtl"(reference=w96) -> ("Pages"=w95:refnum<vi>[])  [unwired: 1 in, 2 out]
                  n50 = for {
                    tunnel: w99 -> [w103]
                    tunnel: w97 -> [_]
                    tunnel: w95 -> [w102] mode=indexing
                    tunnel: w94 -> [w100]
                    n51 = property class="Page"(reference=w102) -> ("ControlsOnPage"=w101:refnum<vi>[])  [unwired: 1 in, 2 out]
                    n52 = for {
                      tunnel: w103 -> [w110]
                      tunnel: w101 -> [w109] mode=indexing
                      tunnel: w100 -> [w104]
                      w108 = refnum<vi> refnum  # Cluster
                      n53 = To More Specific Class(target class=w108, reference=w109) -> (specific class reference=w107:refnum<vi>)  [unwired: 1 in, 1 out]
                      n54 = property class="Clust"(reference=w107) -> ("Label.Text"=w105:string, "Controls[]"=w106:refnum<vi>[])  [unwired: 1 in, 2 out]
                      n55 = for {
                        tunnel: w106 -> [w116] mode=indexing
                        tunnel: w105 -> [w113]
                        tunnel: w110 -> [w112]
                        tunnel: w104 -> [w111]
                        n56 = property class="Ctl"(reference=w116) -> (reference out=w114:refnum<vi>, "ClassName"=w117:string)  [unwired: 1 in, 1 out]
                        n57 = Equal?(x=w117, y="String") -> (x = y?=w115:bool)
                        n58 = case shown="False" w115 {
                          tunnel: w114 -> [w128 w131]
                          tunnel: w113 -> [w122 w130]
                          tunnel: w112 -> [_ w129]
                          tunnel: w111 -> [w121 _]
                          frame False {
                            n59 = Match Pattern(string=w122, regular expression="Channel ") -> (after substring=w125:string)  [unwired: 1 in, 3 out]
                            n60 = Decimal String To Number(string=w125) -> (number=w124:i32)  [unwired: 2 in, 1 out]
                            n61 = Decrement(x=w124) -> (x-1=w120:i32)
                            n62 = Index Array(array=w121, index=w120) -> (element=w119:bool)
                            n63 = Variant To Data(type=variant ("Value"), Variant=w119) -> (data=w126:variant)  [unwired: 1 in, 1 out]
                            n64 = property class="Ctl"(reference=w128, "Value"=w126) -> ()  [unwired: 1 in, 2 out]
                          }
                          frame True {
                            n65 = disable-structure shown="Disabled" {
                              disable-tunnel: w131 -> [w142 _]
                              disable-tunnel: w130 -> [w141 _]
                              disable-tunnel: w129 -> [w137 _]
                              frame Disabled {
                                n66 = Match Pattern(string=w141, regular expression="Channel ") -> (after substring=w139:string)  [unwired: 1 in, 3 out]
                                n67 = Decimal String To Number(string=w139) -> (number=w138:i32)  [unwired: 2 in, 1 out]
                                n68 = Decrement(x=w138) -> (x-1=w136:i32)
                                n69 = Index Array(array=w137, index=w136) -> (element=w135:string)
                                n70 = Variant To Data(type=variant ("Value"), Variant=w135) -> (data=w132:variant, error out=w133:errorcluster)  [unwired: 1 in]
                                n71 = property class="Ctl"(reference=w142, error in=w133, "Value"=w132) -> ()  [unwired: 2 out]
                              }
                              frame Enabled {
                              }
                            }
                          }
                        }
                      }
                    }
                  }
                }
              }
            }
          }
        }
      }
    }
  }
